vi "Create Engine Folder and Copy RT Template.vi"(8 "error in (no error)":errorcluster, 9 "Project Root":path, 10 "Project Name":string, 11 "Inline-Async":refnum<class "NIVS_Inline HW Interface (Inline-Async).lvclass">) -> (0 "error out":errorcluster)   [LabVIEW 2015, in "NIVS_Inline HW Interface (Inline-Async).lvclass"]
uses:
  NIVS_Inline HW Interface (Inline-Async).lvclass
  NIVS_Consolidated_CDW_MetaDataObj/CD Engine lvlib.ctl
  NIVS_Consolidated_CDW_MetaDataObj/Common.ctl
  NIVS_Consolidated_CDW_MetaDataObj/CD Engine lvlib.vi
  NIVS_Consolidated_CDW_MetaDataObj/Common.vi
  NIVS_Consolidated_CDW_MetaDataObj/NIVS_Consolidated_CDW_MetaDataObj.lvclass
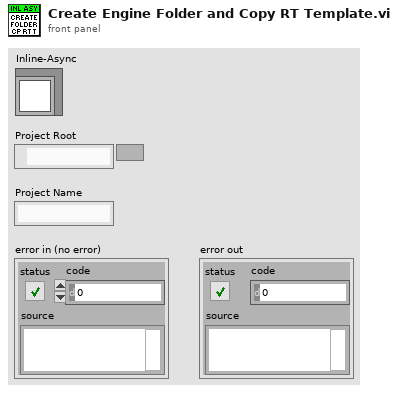
[diagram p1: front panel]
types:
  T1 = typedef "NIVS_Consolidated_CDW_MetaDataObj.lvclass/Common.ctl" = enum16{"ProjectName", "TemplatesFolderName", "ProjectTemplatePathAndName", "TimingAndSyncFolderName", "CustomDeviceFolderName", "PathToTemplates"}
  T2 = typedef "NIVS_Consolidated_CDW_MetaDataObj.lvclass/CD Engine lvlib.ctl" = enum16{"LibraryFileName", "LibraryFolderName", "Engine.FolderName", "Engine.Init.FolderName", "Engine.Run.FolderName", "Engine.Shutdown.FolderName", "Types.FolderName", "Engine.RT Driver VI.TemplatePath", "Engine.RT Driver VI.FileName", "Engine.RTStateVariables.Name", "Engine.RTStateVariables.Name.NoExtension", "Engine.Async.NameExtension", "Engine.Async.TemplateName"}
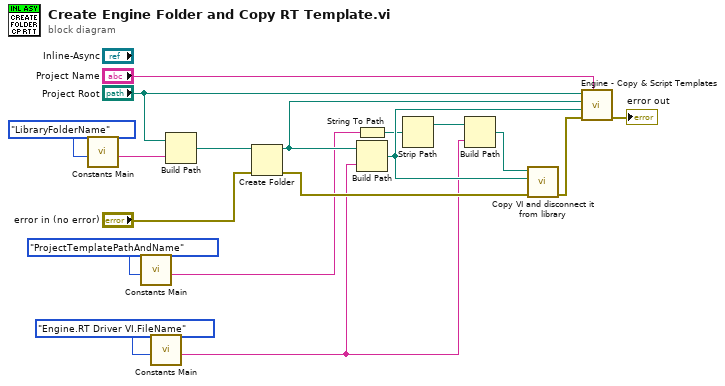
[diagram p0: block diagram]
diagram:
  n1 = call-poly "Constants Main.vi"("Action"=CD_Engine_lvlib."LibraryFolderName") -> ("Output"=w3:string)  [unwired: 10 in]
  n2 = call-poly "Constants Main.vi"("Action"=Common."ProjectTemplatePathAndName") -> ("Output"=w7:string)  [unwired: 10 in]
  n3 = call-poly "Constants Main.vi"("Action"=CD_Engine_lvlib."Engine.RT Driver VI.FileName") -> ("Output"=w8:string)  [unwired: 10 in]
  n4 = Build Path(base path="Project Root", name or relative path=w3) -> (appended path=w1:path)
  n5 = Create Folder(path (use dialog)=w1, error in="error in (no error)") -> (created path=w14:path, error out=w16:errorcluster)  [unwired: 1 in, 1 out]
  n6 = String To Path(string=w7) -> (path=w6:path)
  n7 = Build Path(base path=w14, name or relative path=w8) -> (appended path=w13:path)
  n8 = Strip Path(path=w6) -> (stripped path=w10:path)  [unwired: 1 out]
  n9 = Build Path(base path=w10, name or relative path=w8) -> (appended path=w5:path)
  n10 = call "Copy VI and disconnect it from library.vi"("error in (no error)"=w16, "VI Target Path"=w13, "VI Source Path"=w5) -> ("error out"=w11:errorcluster)  [unwired: 8 in]
  n11 = call "Engine - Copy & Script Templates.vi"("CD Name"="Project Name", "error in (no error)"=w11, "RT Driver VI Path"=w13, "RT Driver Folder Path"=w14, "CD Source Folder Path"="Project Root") -> ("error out"=→"error out":errorcluster)  [unwired: 6 in]
